vi "Version_Conversion_Data.vi"(8 "Error In":errorcluster, 10 "Version In":string) -> (0 "Error Out":errorcluster, 2 "Version Out":string)   [LabVIEW 2021]
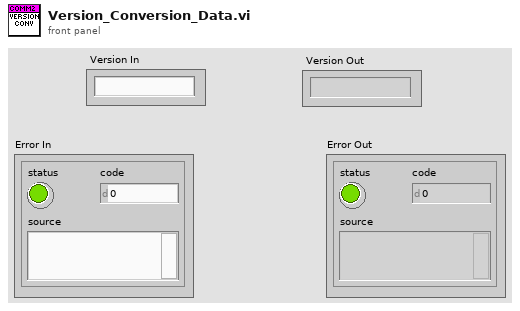
[diagram p1: front panel]
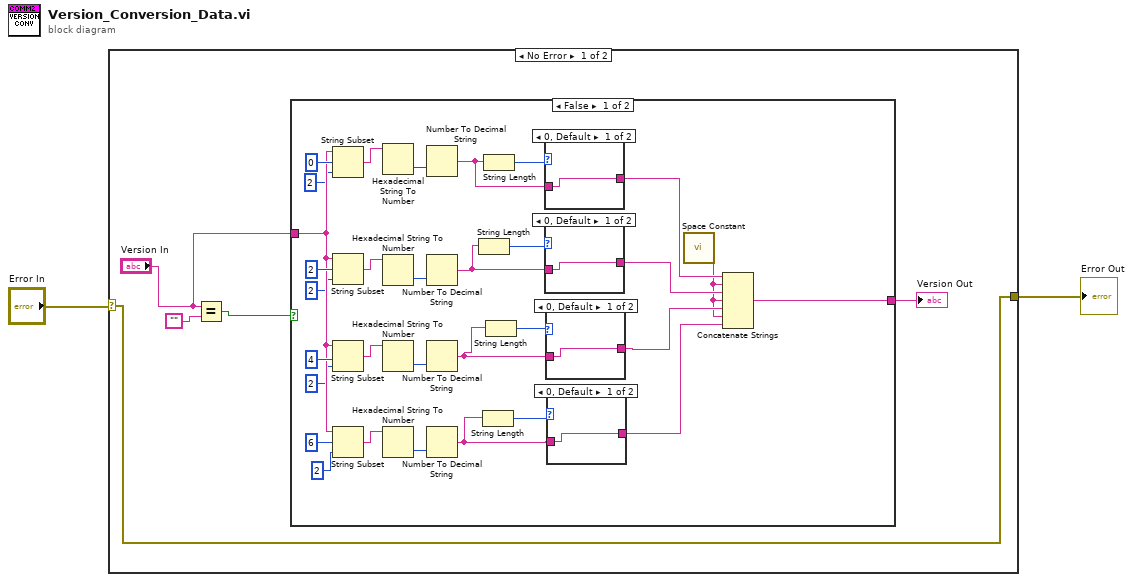
[diagram p0: block diagram]
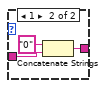
[diagram p2: hidden frame]
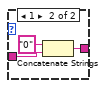
[diagram p3: hidden frame]
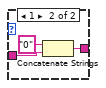
[diagram p4: hidden frame]
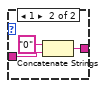
[diagram p5: hidden frame]
diagram:
  n1 = case shown="No Error" "Error In" {
    selector: "Error In" -> [w3 w56]
    tunnel: [w3 w56] -> w1
    frame No Error {
      n2 = Equal?(x="Version In", y="") -> (x = y?=w6:bool)
      n3 = case shown="False" w6 {
        tunnel: "Version In" -> [w13 w55]
        tunnel: [w12 w55] -> w4
        frame False {
          n4 = String Subset(string=w13, offset (0)=0 ("length (rest)"), length (rest)=2 ("length (rest)")) -> (substring=w36:string)
          n5 = String Subset(string=w13, offset (0)=2 ("length (rest)"), length (rest)=2 ("length (rest)")) -> (substring=w35:string)
          n6 = String Subset(string=w13, offset (0)=4, length (rest)=2 ("length (rest)")) -> (substring=w32:string)
          n7 = String Subset(string=w13, offset (0)=6, length (rest)=2 ("length (rest)")) -> (substring=w31:string)
          n8 = Hexadecimal String To Number(string=w36) -> (number=w34:u32)  [unwired: 2 in, 1 out]
          n9 = Hexadecimal String To Number(string=w35) -> (number=w33:u32)  [unwired: 2 in, 1 out]
          n10 = Hexadecimal String To Number(string=w32) -> (number=w30:u32)  [unwired: 2 in, 1 out]
          n11 = Hexadecimal String To Number(string=w31) -> (number=w27:u32)  [unwired: 2 in, 1 out]
          n12 = Number To Decimal String(number=w34) -> (decimal integer string=w25:string)  [unwired: 1 in]
          n13 = Number To Decimal String(number=w33) -> (decimal integer string=w19:string)  [unwired: 1 in]
          n14 = Number To Decimal String(number=w30) -> (decimal integer string=w21:string)  [unwired: 1 in]
          n15 = Number To Decimal String(number=w27) -> (decimal integer string=w22:string)  [unwired: 1 in]
          n16 = String Length(string=w19) -> (length=w20:i32)
          n17 = String Length(string=w22) -> (length=w23:i32)
          n18 = String Length(string=w25) -> (length=w26:i32)
          n19 = String Length(string=w21) -> (length=w24:i32)
          n20 = case shown="0, Default" w26 {
            tunnel: w25 -> [w51 w53]
            tunnel: [w51 w52] -> w18
            frame 0, Default {
            }
            frame 1 {
              n21 = Concatenate Strings("0" ("string"), w53) -> (w52:string)
            }
          }
          n22 = case shown="0, Default" w20 {
            tunnel: [w47 w49] -> w17
            tunnel: w19 -> [w47 w48]
            frame 0, Default {
            }
            frame 1 {
              n23 = Concatenate Strings("0" ("string"), w48) -> (w49:string)
            }
          }
          n24 = case shown="0, Default" w24 {
            tunnel: w21 -> [w43 w45]
            tunnel: [w43 w44] -> w16
            frame 0, Default {
            }
            frame 1 {
              n25 = Concatenate Strings("0" ("string"), w45) -> (w44:string)
            }
          }
          n26 = case shown="0, Default" w23 {
            tunnel: w22 -> [w39 w41]
            tunnel: [w39 w40] -> w15
            frame 0, Default {
            }
            frame 1 {
              n27 = Concatenate Strings("0" ("string"), w41) -> (w40:string)
            }
          }
          n28 = call <vilib>:"Space Constant.vi"() -> ("String"=w14:string)
          n29 = Concatenate Strings(w18, w14, w17, w14, w16, w14, w15) -> (w12:string)
        }
        frame True {
        }
      }
      "Version Out" <- w4
    }
    frame Error {
    }
  }
  "Error Out" <- w1
